vi "User Event-Undock-Value Change.vi"(8 "Error In":errorcluster, 11 "Appearance Actor in":refnum<class "Appearance Actor.lvclass">) -> (0 "Error Out":errorcluster, 3 "Appearance Actor out":refnum<class "Appearance Actor.lvclass">)   [LabVIEW 2021, in "Appearance Actor.lvlib" / "Appearance Actor.lvclass"]
doc: "Handles Undock Event. By Default, undocks (or docks if undocked) the FP if possible. Override this method to change its behavior."
uses:
  Appearance Actor.lvclass
  C:/Program Files (x86)/National Instruments/LabVIEW 2021/vi.lib/ActorFramework/Actor/Actor.lvclass
  <vilib>/ActorFramework/Actor/Actor.lvclass/Actor.ctl
  <vilib>/ActorFramework/Message Enqueuer/Message Enqueuer.lvclass/Message Enqueuer.ctl
  Appearance Actor.lvclass/Appearance Actor.ctl
  Typedefs/Docking State--enum.ctl
  <vilib>/ActorFramework/Message Enqueuer/Init from Existing Queue.vi
  <vilib>/MGI/Panel Manager/Panel/Panel/Subpanel/Subpanel.lvclass
  C:/Program Files (x86)/National Instruments/LabVIEW 2021/vi.lib/MGI/Panel Manager/Panel/Panel/Panel.lvclass
  <vilib>/MGI/Panel Manager/Panel/Panel/Window/Window.lvclass
  <vilib>/MGI/Panel Manager/Panel/Panel/Subpanel/Subpanel.vi
  <vilib>/MGI/Panel Manager/Panel/Panel/Window/Window.vi
  <vilib>/ActorFramework/Message Enqueuer/Message Enqueuer.lvclass
  <vilib>/ActorFramework/Actor/Actor.lvclass
  <vilib>/MGI/Panel Manager/Panel Actor/Panel Actor Messages/Change Panel Msg/Change Panel Msg.lvclass
  <vilib>/MGI/Panel Manager/Panel/Panel.lvlib
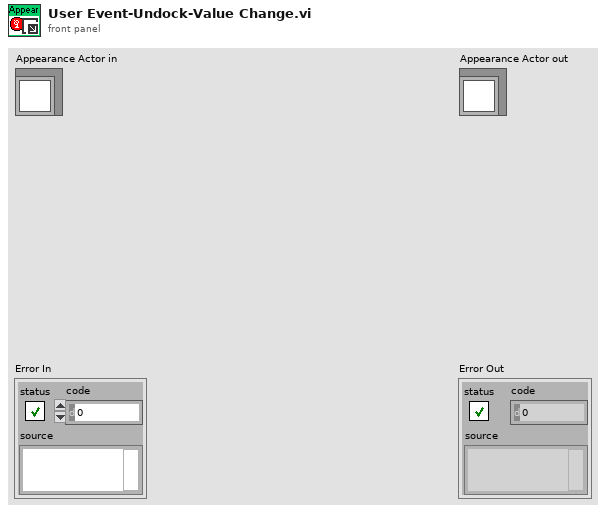
[diagram p1: front panel]
types:
  T1 = typedef "Appearance Actor.lvlib/Appearance Actor.lvclass/Docking State--enum.ctl" = enum16{"Not A SubPanel", "Docked", "UnDocked"}
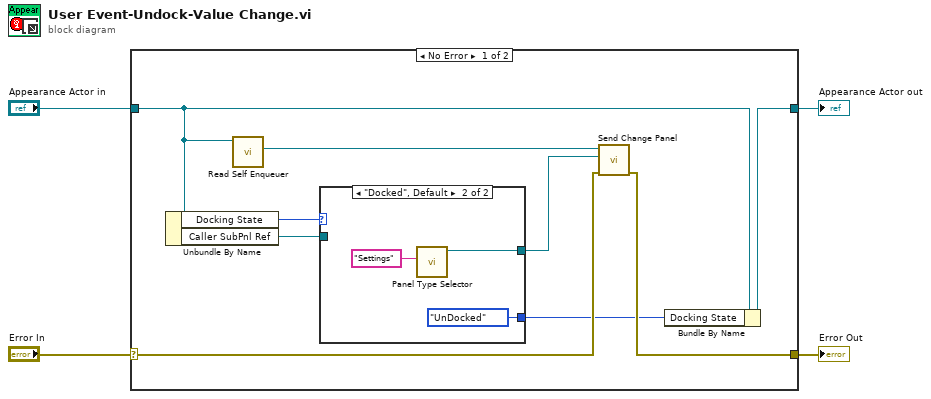
[diagram p0: block diagram]
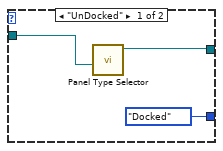
[diagram p2: hidden frame]
diagram:
  n1 = case shown="No Error" "Error In" {
    selector: "Error In" -> [w11 w21]
    tunnel: [w10 w21] -> w3
    tunnel: [w6 w20] -> w1
    tunnel: "Appearance Actor in" -> [w9 w20]
    frame No Error {
      n2 = Unbundle By Name(w9) -> ("Docking State"=w8:T1, "Caller SubPnl Ref"=w7:refnum<vi>)
      n3 = call <vilib>:"Read Self Enqueuer.vi"("Actor"=w9) -> ("Self Enqueuer"=w13:refnum<class "Message Enqueuer.lvclass">)  [unwired: 10 in]
      n4 = case shown="\"Docked\", Default" w8 {
        tunnel: [w16 w18] -> w12
        tunnel: w7 -> [w15 _]
        tunnel: [Docking_State--enum."Docked" ("Docking State") Docking_State--enum."UnDocked" ("Docking State")] -> w5
        frame "UnDocked" {
          n5 = call-poly <vilib>:"Panel Type Selector.vi"("Sub Panel"=w15) -> ("Subpanel Out"=w16:refnum<class "Subpanel.lvclass">)  [unwired: 9 in, 1 out]
        }
        frame "Docked", Default {
          n6 = call-poly <vilib>:"Panel Type Selector.vi"("Default Title"="Settings") -> ("Window out"=w18:refnum<class "Window.lvclass">)  [unwired: 9 in, 1 out]
        }
      }
      n7 = call <vilib>:"Send Change Panel.vi"("error in (no error)"=w11, "New Panel"=w12, "Message Enqueuer in"=w13) -> ("error out"=w10:errorcluster)  [unwired: 7 in, 1 out]
      n8 = Bundle By Name(cluster=w9, "Docking State"=w5) -> (w6:refnum<class "Appearance Actor.lvclass">)
    }
    frame Error {
    }
  }
  "Error Out" <- w3
  "Appearance Actor out" <- w1
